vi "Get gRPC Device Location.vi"(8 "error in":errorcluster, 10 "provided_interface":string, 11 "discovery service gRPC ID":T1) -> (0 "error out":errorcluster, 2 "gRPC device location":T2, 3 "discovery service gRPC ID out":T1)   [LabVIEW 2020, in "Measurement Service Helpers.lvlib"]
doc: "Gets the location of the gRPC device server based on the provided interface."
uses:
  Measurement Service Helpers.lvlib
  <vilib>/MeasurementLink/MeasurementLink Discovery Client/RPC Messages/ni_measurementlink_discovery_v1_ServiceLocation.ctl
  <vilib>/gRPC/LabVIEW gRPC Library/Shared/grpcId.ctl
  <vilib>/MeasurementLink/MeasurementLink Discovery Client/RPC Messages/ni_measurementlink_discovery_v1_ResolveServiceRequest.ctl
  <vilib>/MeasurementLink/MeasurementLink Discovery Client/MeasurementLink Discovery Client.lvlib
  <vilib>/gRPC/LabVIEW gRPC Library/grpc-lvsupport-release.lvlib
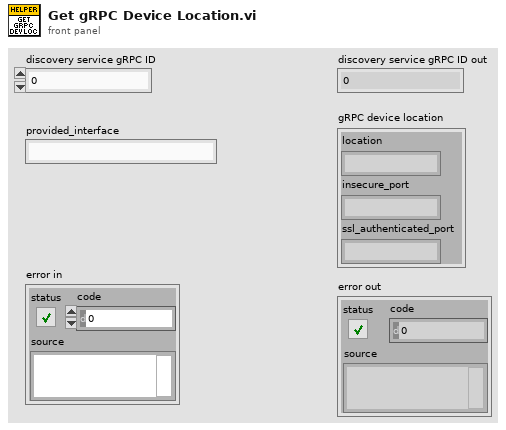
[diagram p1: front panel]
types:
  T1 = typedef "grpc-lvsupport-release.lvlib/grpcId.ctl" = u64
  T2 = typedef "MeasurementLink Discovery Client.lvlib/ni_measurementlink_discovery_v1_ServiceLocation.ctl" = cluster{"location":string, "insecure_port":string, "ssl_authenticated_port":string}
  T3 = typedef "MeasurementLink Discovery Client.lvlib/ni_measurementlink_discovery_v1_ResolveServiceRequest.ctl" = cluster{"provided_interface":string, "service_class":string}
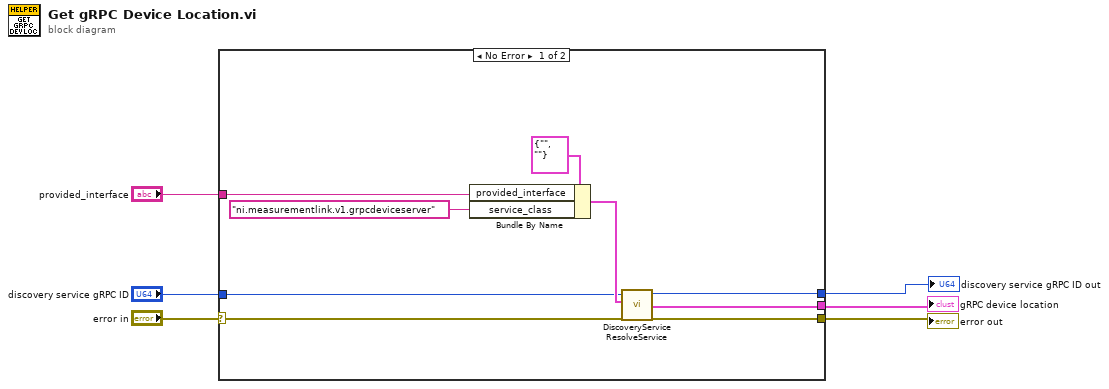
[diagram p0: block diagram]
diagram:
  n1 = case shown="No Error" "error in" {
    selector: "error in" -> [w15 w17]
    tunnel: [w14 w17] -> w5
    tunnel: [w13 _] -> w4
    tunnel: "provided_interface" -> [w10 _]
    tunnel: "discovery service gRPC ID" -> [w8 w16]
    tunnel: [w7 w16] -> w1
    frame No Error {
      n2 = Bundle By Name(cluster=T3 {"provided_interface"="", "service_class"=""} ("Request Data"), "provided_interface"=w10, "service_class"="ni.measurementlink.v1.grpcdeviceserver") -> (w9:T3)
      n3 = call <vilib>:"DiscoveryService ResolveService.vi"("error in"=w15, "Request Data"=w9, "gRPC ID"=w8) -> ("error out"=w14:errorcluster, "Response Data"=w13:T2, "gRPC ID out"=w7:T1)  [unwired: 6 in]
    }
    frame Error {
    }
  }
  "error out" <- w5
  "gRPC device location" <- w4
  "discovery service gRPC ID out" <- w1
